vi "Write Global Error Manager Spawned flag.vi"(8 "error in (no error)":errorcluster, 10 "Status":bool, 11 "Error Manager in":refnum<class "Local Error Manager.lvclass">) -> (0 "error out":errorcluster, 3 "Error Manager out":refnum<class "Local Error Manager.lvclass">)   [LabVIEW 2020, in "TALOS.lvlib" / "Error Manager.lvlib" / "Local Error Manager.lvclass"]
uses:
  Local Error Manager/Local Error Manager.lvclass
  Local Error Manager/Local Error Manager.lvclass/Local Error Manager.ctl
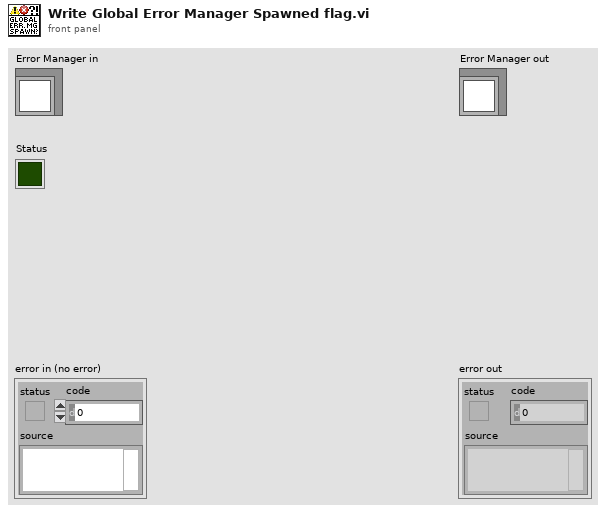
[diagram p1: front panel]
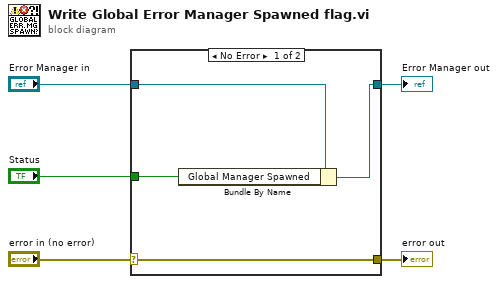
[diagram p0: block diagram]
diagram:
  n1 = case shown="No Error" "error in (no error)" {
    selector: "error in (no error)" -> [w9 w10]
    tunnel: [w9 w10] -> w4
    tunnel: [w7 w11] -> w2
    tunnel: "Error Manager in" -> [w8 w11]
    tunnel: "Status" -> [w6 _]
    frame No Error {
      n2 = Bundle By Name(cluster=w8, "Global Manager Spawned"=w6) -> (w7:refnum<class "Local Error Manager.lvclass">)
    }
    frame Error {
    }
  }
  "error out" <- w4
  "Error Manager out" <- w2
